vi "score generator.vi"(5 "min score":dbl=20.0, 6 "max score":dbl=80.0) -> (2 "generated score":dbl)   [LabVIEW 2014]
doc: "Which can generate a random score number between the minmium and maximum score values given from the inputs."
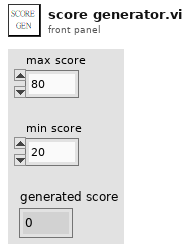
[diagram p1: front panel]
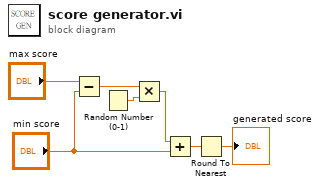
[diagram p0: block diagram]
diagram:
  n1 = Subtract(x="max score", y="min score") -> (x-y=w5:dbl)
  n2 = Random Number (0-1)() -> (number: 0 to 1=w4:dbl)
  n3 = Multiply(x=w5, y=w4) -> (x*y=w6:dbl)
  n4 = Add(x=w6, y="min score") -> (x+y=w7:dbl)
  n5 = Round To Nearest(number=w7) -> (nearest integer value=→"generated score":dbl)
